vi "IntakeNetwork.vi"(8 "error in (no error)":errorcluster) -> (0 "error out":errorcluster)   [LabVIEW 2023]
doc: "Writes motor demand and sensor data to the Dashboard."
uses:
  IntakeGlobal.vi
  <vilib>/Rock Robotics/Network Tables/NT Write Boolean.vi
  <vilib>/Rock Robotics/Network Tables/NT Write Number.vi
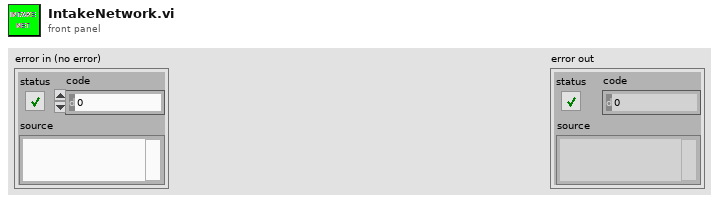
[diagram p1: front panel]
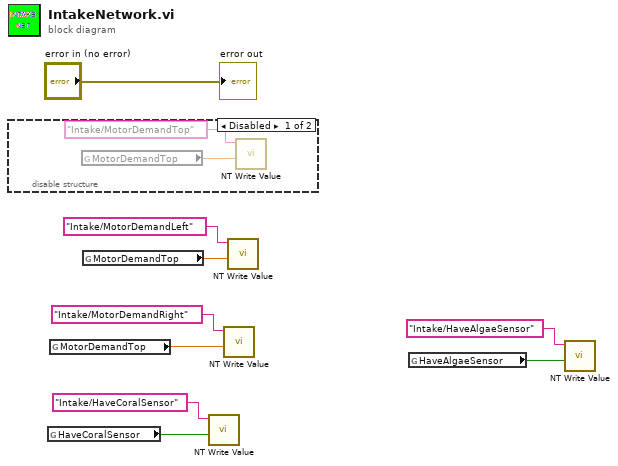
[diagram p0: block diagram]
diagram:
  n1 = disable-structure shown="Disabled" {
    frame Disabled {
      n2 = global read "IntakeGlobal.vi" "MotorDemandTop"() -> (w10:dbl)
      n3 = call-poly <vilib>:"NT Write Value.vi"("value"=w10, "name"="Intake/MotorDemandTop") -> ()  [unwired: 9 in, 1 out]
    }
    frame Enabled {
    }
  }
  n4 = global read "IntakeGlobal.vi" "HaveCoralSensor"() -> (w1:bool)
  n5 = global read "IntakeGlobal.vi" "MotorDemandTop"() -> (w2:dbl)
  n6 = global read "IntakeGlobal.vi" "MotorDemandTop"() -> (w3:dbl)
  n7 = call-poly <vilib>:"NT Write Value.vi"("value"=w1, "name"="Intake/HaveCoralSensor") -> ()  [unwired: 9 in, 1 out]
  n8 = call-poly <vilib>:"NT Write Value.vi"("value"=w2, "name"="Intake/MotorDemandRight") -> ()  [unwired: 9 in, 1 out]
  n9 = call-poly <vilib>:"NT Write Value.vi"("value"=w3, "name"="Intake/MotorDemandLeft") -> ()  [unwired: 9 in, 1 out]
  n10 = global read "IntakeGlobal.vi" "HaveAlgaeSensor"() -> (w4:bool)
  n11 = call-poly <vilib>:"NT Write Value.vi"("value"=w4, "name"="Intake/HaveAlgaeSensor") -> ()  [unwired: 9 in, 1 out]
  "error out" <- "error in (no error)"
